vi "Split Registers by Direction.vi"(7 "Group":bool, 8 "error in":errorcluster, 11 "vi info":T1 {"RegisterMap"."Address" format="%.0x"}) -> (0 "error out":errorcluster, 2 "Controls":T8[](array[typedef]) {"Data Type" format="%.0x"}, 3 "Indicator":T8[](array[typedef]) {"Data Type" format="%.0x"})   [LabVIEW 2018, in "FPGA Addon System Explorer.lvlib"]
uses:
  FPGA Addon System Explorer.lvlib
  Addon Shared/Types/Register Information.ctl
  Addon Shared/Types/Data Type.ctl
  <vilib>/rvi/Bitfile/niFpgaBitfileStructure_VI.ctl
  <vilib>/rvi/Bitfile/nirviControlStructure.ctl
  <vilib>/rvi/Bitfile/nirviTypdefDescription.ctl
  <vilib>/rvi/Bitfile/nirviMechanicalAction.ctl
  <vilib>/rvi/Bitfile/nirviSubControlStructure.ctl
  <vilib>/rvi/Bitfile/nirviClusterElementControl.ctl
  <vilib>/picture/picture.llb/imagedata.ctl
  niveristand-fpga-addon-speciality-io/Source/Types/PWM.Measure.Analog.Measurement.ctl
  niveristand-fpga-addon-speciality-io/Source/Types/PWM.Measure.Digital.Measurement.ctl
  niveristand-fpga-addon-speciality-io/Source/Types/Static.Measure.Digital.Measurement.ctl
  niveristand-fpga-addon-speciality-io/Source/Types/QuadratureEncoder.Measure.Digital.Measurement.ctl
  niveristand-fpga-addon-speciality-io/Source/Types/PWM.Generate.Digital.Settings.ctl
  niveristand-fpga-addon-speciality-io/Source/Types/PWM.Measure.Analog.Settings.ctl
  niveristand-fpga-addon-speciality-io/Source/Types/PWM.Measure.Digital.Settings.ctl
  niveristand-fpga-addon-speciality-io/Source/Types/Sine.Generate.Settings.ctl
  niveristand-fpga-addon-speciality-io/Source/Types/Static.Generate.Digital.Settings.ctl
  niveristand-fpga-addon-speciality-io/Source/Types/Static.Measure.Digital.Settings.ctl
  niveristand-fpga-addon-speciality-io/Source/Types/WSS.Generate.Digital.Settings.ctl
  niveristand-fpga-addon-speciality-io/Source/Types/QuadratureEncoder.Measure.Digital.Settings.ctl
  Addon Shared/FPGA Addon Shared.lvlib
  niveristand-fpga-addon-speciality-io/Source/Speciality FPGA IO.lvlib
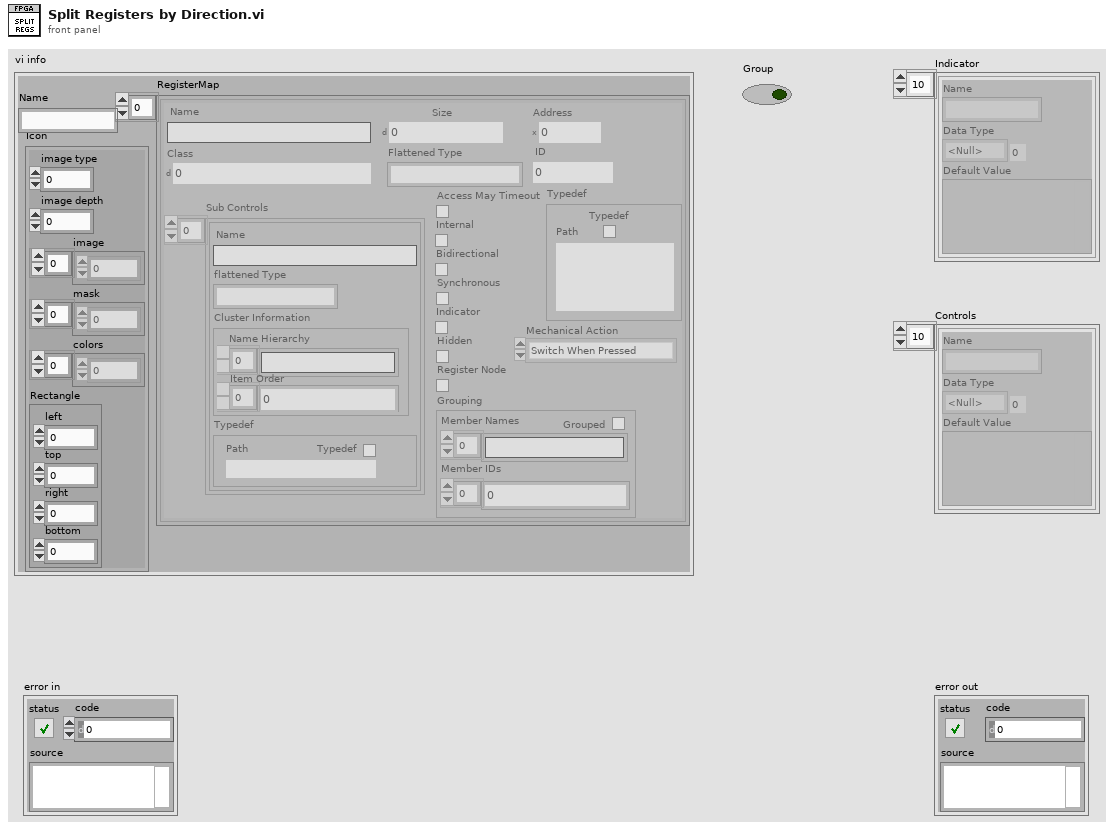
[diagram p1: front panel]
types:
  T1 = typedef "niFpgaBitfileStructure_VI.ctl" = cluster{"Name":string, "RegisterMap":T2[], "Icon":T7}
  T2 = typedef "nirviControlStructure.ctl" = cluster{"Name":string, "Hidden":bool, "Indicator":bool, "Flattened Type":string, "Grouping":cluster{"Grouped":bool, "Member Names":string[], "Member IDs":u32[]}, "Address":u32, "Size":u32, "Class":u32, "Internal":bool, "Typedef":T3, "ID":u32, "Bidirectional":bool, "Synchronous":bool, "Mechanical Action":T4, "Sub Controls":T5[], "Access May Timeout":bool, "Register Node":bool}
  T3 = typedef "nirviTypdefDescription.ctl" = cluster{"Typedef":bool, "Path":path}
  T4 = typedef "nirviMechanicalAction.ctl" = enum8{"Switch When Pressed", "Switch When Released", "Switch Until Released", "Latch When Pressed", "Latch When Released", "Latch Until Released"}
  T5 = typedef "nirviSubControlStructure.ctl" = cluster{"Name":string, "flattened Type":string, "Cluster Information":T6, "Typedef":T3}
  T6 = typedef "nirviClusterElementControl.ctl" = cluster{"Name Hierarchy":string[], "Item Order":u32[]}
  T7 = typedef "imagedata.ctl" = cluster{"image type":i32, "image depth":i32, "image":u8[], "mask":u8[], "colors":u32[], "Rectangle":cluster{"left":i16, "top":i16, "right":i16, "bottom":i16}}
  T8 = typedef "FPGA Addon Shared.lvlib/Register Information.ctl" = cluster{"Name":string, "Data Type":T9, "Default Value":variant}
  T9 = typedef "FPGA Addon Shared.lvlib/Data Type.ctl" = enum8{"<Null>", "I8", "I16", "I32", "I64", "U8", "U16", "U32", "U64", "SGL", "Boolean", "Analog PWM In Settings", "Analog PWM In", "Digital PWM In Settings", "Digital PWM In", "Digital PWM Out", "Sine Out", "FXP+/-24.5", "FXP+/-16.5", "FXP+/-32.8", "FXP+/-64.32", "FXP+/-16.7", "FXP+/-20.5", "FXP+/-27.5", "FXP+/-32.16", "FXP+16.3", "FXP+18.3", "Digital Static In", "Digital Static Out", "Digital Static In Settings", "Digital WSS Out", "Quad Encoder Settings", "Quad Encoder In", "Group"}
  T10 = typedef "Speciality FPGA IO.lvlib/QuadratureEncoder.Measure.Digital.Measurement.ctl" = cluster{"POSITION":i32}
  T11 = typedef "Speciality FPGA IO.lvlib/Static.Measure.Digital.Measurement.ctl" = cluster{"STATE":bool}
  T12 = typedef "Speciality FPGA IO.lvlib/PWM.Measure.Digital.Measurement.ctl" = cluster{"ACTIVE TICKS":u32, "INACTIVE TICKS":u32, "ACQ TICKS":u32}
  T13 = typedef "Speciality FPGA IO.lvlib/PWM.Measure.Analog.Measurement.ctl" = cluster{"ACTIVE TICKS":u32, "INACTIVE TICKS":u32, "ACQ TICKS":u32, "ACTIVE VOLTAGE":fxp<+/-,32,8>, "INACTIVE VOLTAGE":fxp<+/-,32,8>}
  T14 = typedef "Speciality FPGA IO.lvlib/QuadratureEncoder.Measure.Digital.Settings.ctl" = cluster{"DIRECTION":u8, "RESET VALUE":i32, "A RESET STATE":bool, "B RESET STATE":bool, "Z RESET STATE":bool}
  T15 = typedef "Speciality FPGA IO.lvlib/WSS.Generate.Digital.Settings.ctl" = cluster{"ACTIVE EDGE":bool, "ACTIVE TICKS":u32, "INACTIVE TICKS":u32, "DATA":u8, "SENSOR TYPE":u8}
  T16 = typedef "Speciality FPGA IO.lvlib/Static.Measure.Digital.Settings.ctl" = cluster{"ACTIVE EDGE":bool}
  T17 = typedef "Speciality FPGA IO.lvlib/Static.Generate.Digital.Settings.ctl" = cluster{"ACTIVE EDGE":bool, "OUTPUT":bool}
  T18 = typedef "Speciality FPGA IO.lvlib/Sine.Generate.Settings.ctl" = cluster{"AMP":fxp<+/-,32,8>, "OFFSET":fxp<+/-,32,8>, "PERIODS/TICKS":fxp<+,32,0>}
  T19 = typedef "Speciality FPGA IO.lvlib/PWM.Measure.Digital.Settings.ctl" = cluster{"ACTIVE EDGE":bool, "TIMEOUT":u32}
  T20 = typedef "Speciality FPGA IO.lvlib/PWM.Measure.Analog.Settings.ctl" = cluster{"ACTIVE EDGE":bool, "TIMEOUT":u32, "THRESHOLD":fxp<+/-,32,8>}
  T21 = typedef "Speciality FPGA IO.lvlib/PWM.Generate.Digital.Settings.ctl" = cluster{"ACTIVE EDGE":bool, "ACTIVE TICKS":u32, "INACTIVE TICKS":u32}
  T22 = typedef "Type Descriptor Enumeration__ogtk.ctl" = enum8{"<Null>", "I8", "I16", "I32", "I64", "U8", "U16", "U32", "U64", "SGL", "DBL", "EXT", "CSG", "CDB", "CXT", "0x0F", "0x10", "0x11", "0x12", "0x13", "0x14", "Enum U8", "Enum U16", "Enum U32", "Enum U64", "SGL PQ", "DBL PQ", "EXT PQ", "CSG PQ", "CDB PQ", "CXT PQ", "0x1F", "0x20", "Boolean", "0x22", "0x23", "0x24", "0x25", "0x26", "0x27", "0x28", "0x29", "0x2A", "0x2B", "0x2C", "0x2D", "0x2E", "0x2F", "String", "0x31", "Path", "Pict", "0x34", "0x35", "0x36", "DAQ", "0x38", "0x39", "0x3A", "0x3B", "0x3C", "0x3D", "0x3E", "0x3F", "Array", "0x41", "0x42", "0x43", "0x44", "0x45", "0x46", "0x47", "0x48", "0x49", "0x4A", "0x4B", "0x4C", "0x4D", "0x4E", "0x4F", "Cluster", "0x51", "0x52", "Variant", "Waveform", "0x55", "0x56", "0x57", "0x58", "0x59", "0x5A", "0x5B", "0x5C", "0x5D", "0x5E", "0x5F", "0x60", "0x61", "0x62", "0x63", "0x64", "0x65", "0x66", "0x67", "0x68", "0x69", "0x6A", "0x6B", "0x6C", "0x6D", "0x6E", "0x6F", "Refnum"}
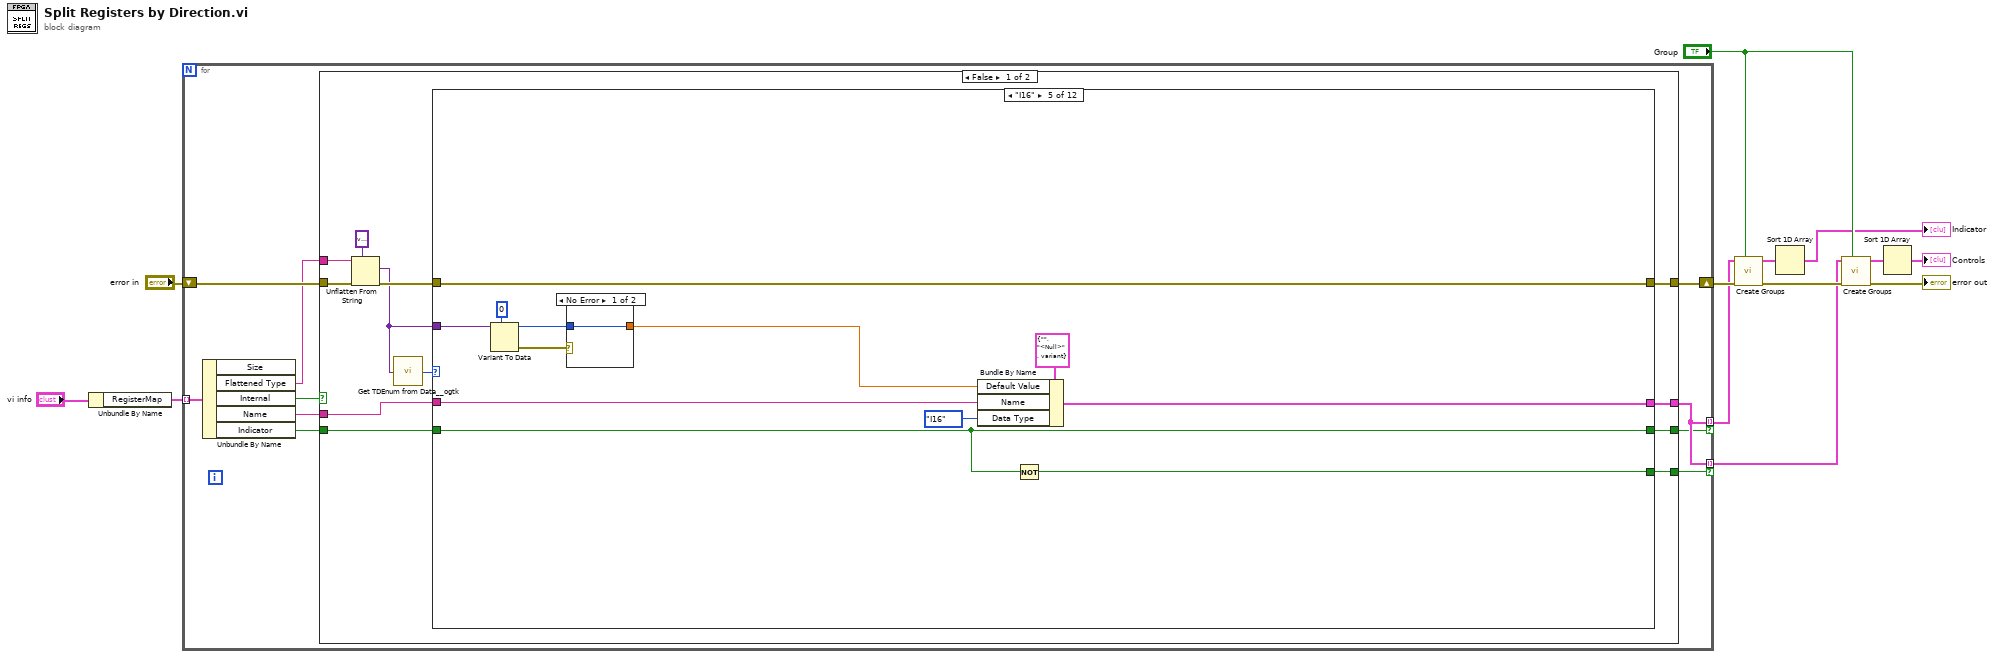
[diagram p0: block diagram]
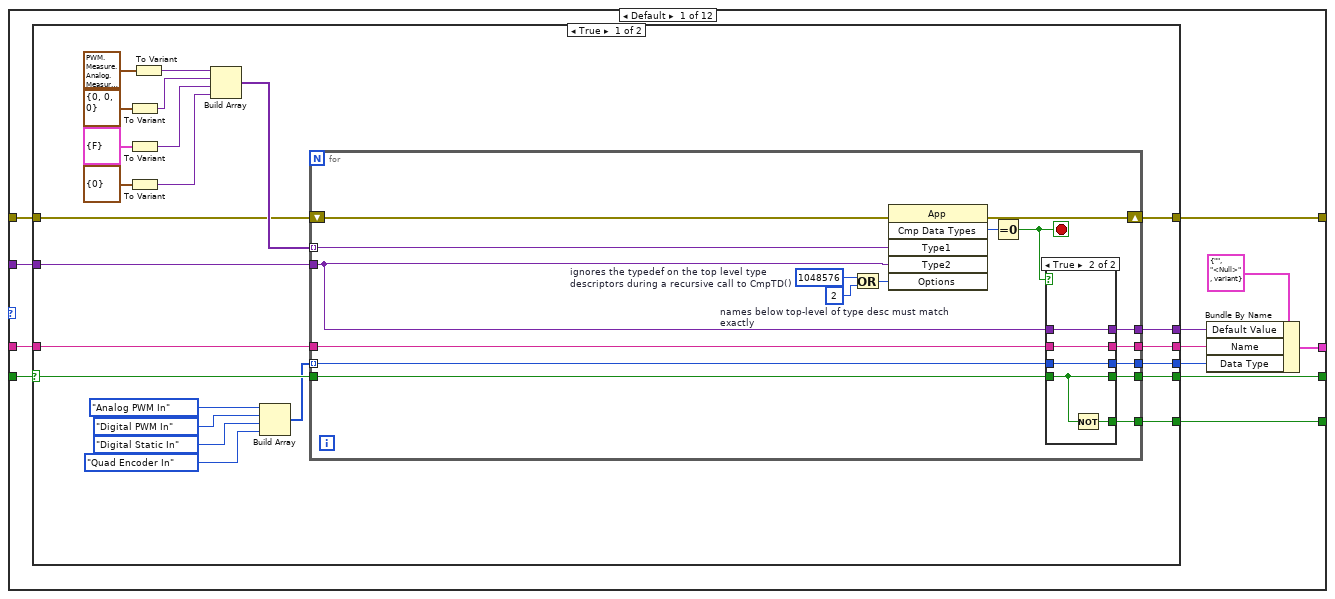
[diagram p2: hidden frame]
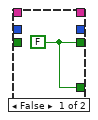
[diagram p3: hidden frame]
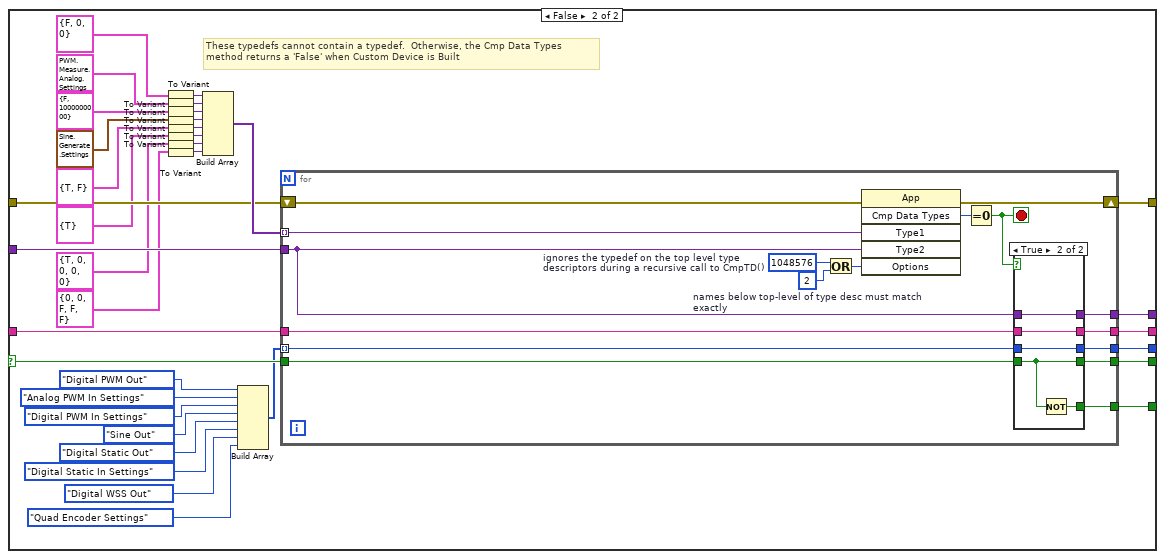
[diagram p4: hidden frame]
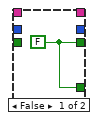
[diagram p5: hidden frame]
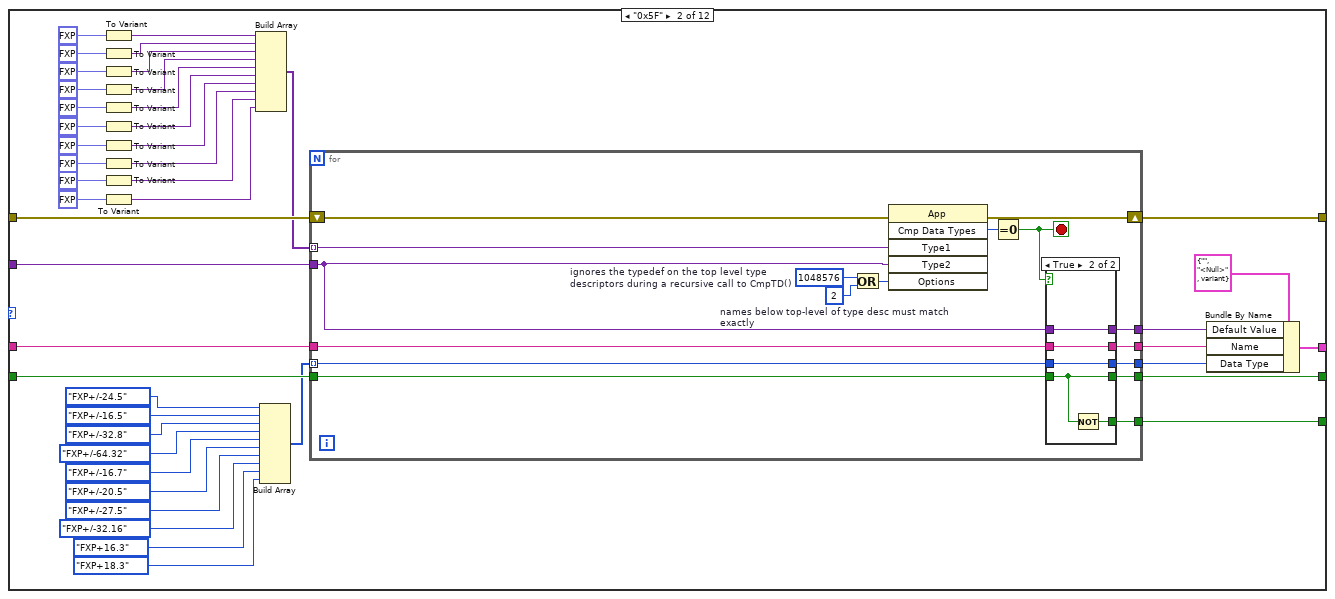
[diagram p6: hidden frame]
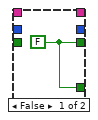
[diagram p7: hidden frame]
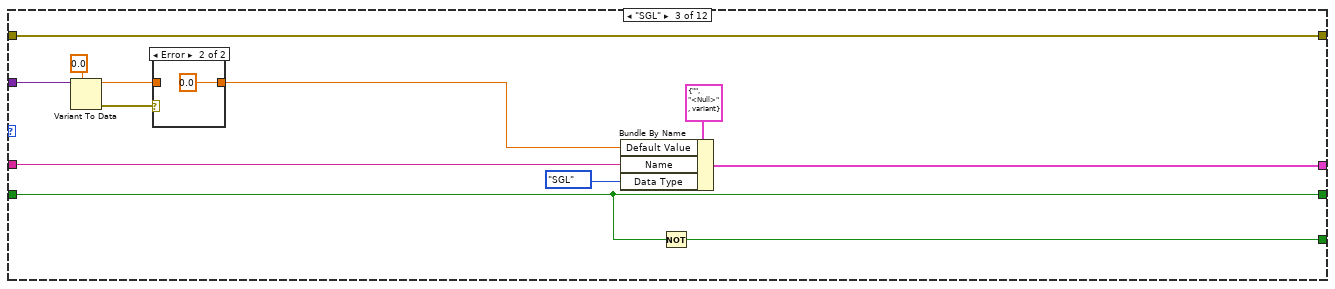
[diagram p8: hidden frame]
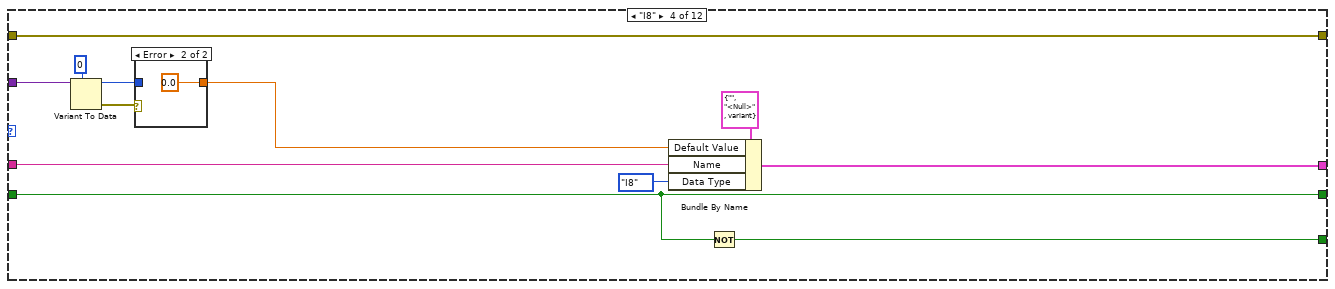
[diagram p10: hidden frame]
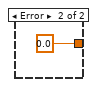
[diagram p12: hidden frame]
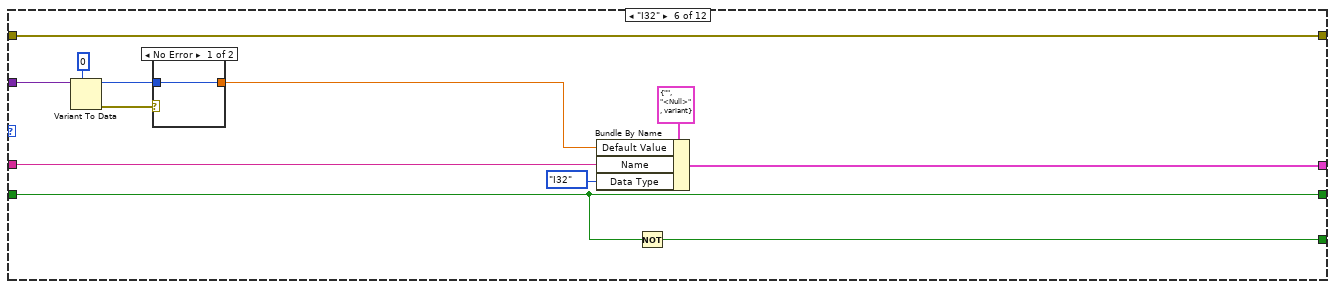
[diagram p13: hidden frame]
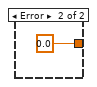
[diagram p14: hidden frame]
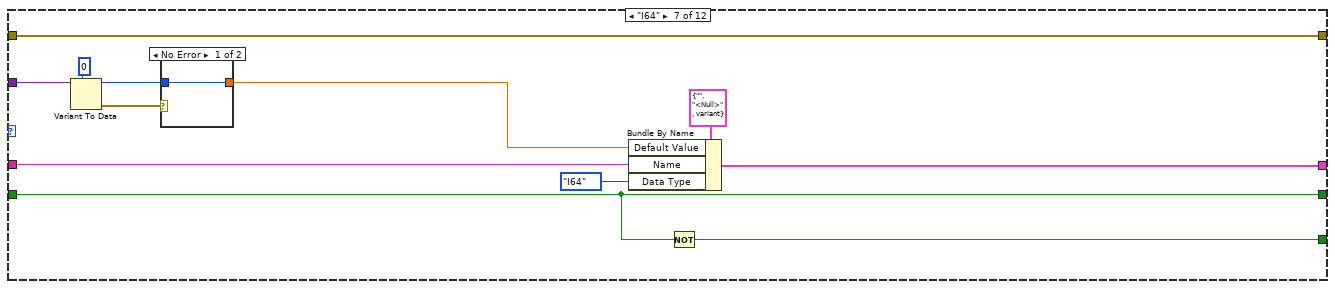
[diagram p15: hidden frame]
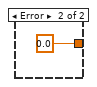
[diagram p16: hidden frame]
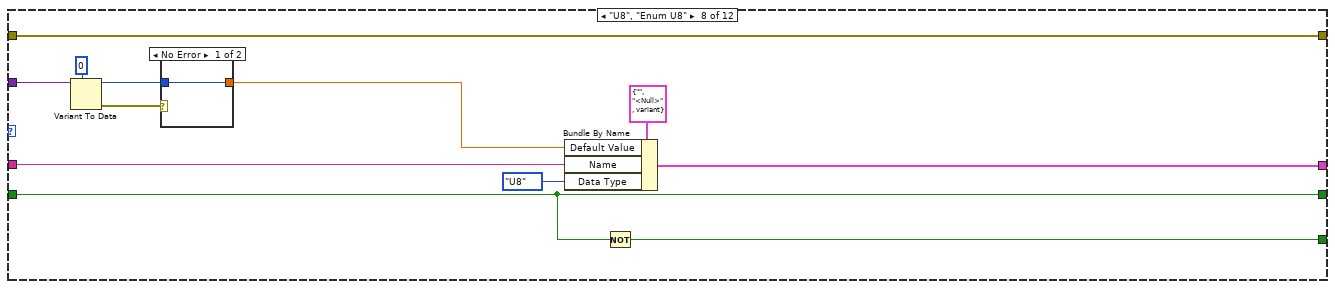
[diagram p17: hidden frame]
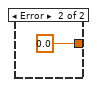
[diagram p18: hidden frame]
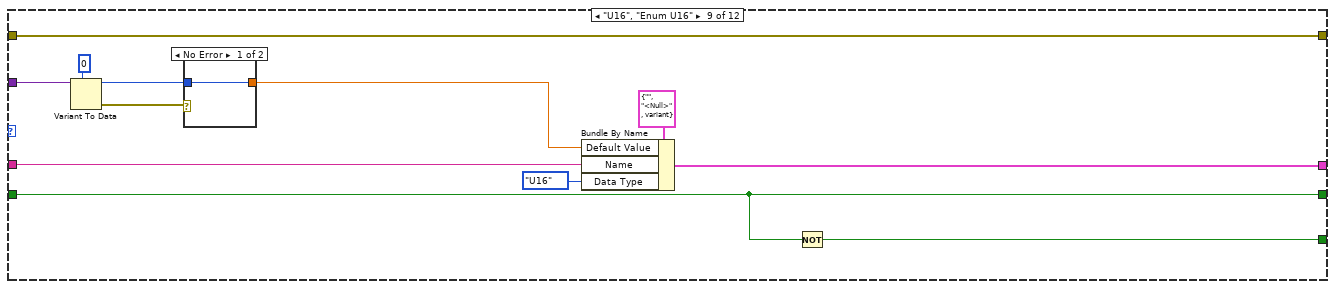
[diagram p19: hidden frame]
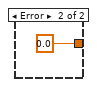
[diagram p20: hidden frame]
diagram:
  n1 = Unbundle By Name("vi info") -> ("RegisterMap"=w13:T2[])
  n2 = for {
    tunnel: w13 -> [w18] mode=indexing
    tunnel: [w23] -> w6 mode=indexing if=w22
    tunnel: [w23] -> w5 mode=indexing if=w21
    shift-right: [w20] -> w10
    shift-left: "error in" -> [w19]
    n3 = Unbundle By Name(w18) -> ("Flattened Type"=w14:string, "Internal"=w15:bool, "Name"=w16:string, "Indicator"=w17:bool)  [unwired: 1 out]
    n4 = case shown="False" w15 {
      tunnel: w16 -> [w34 _]
      tunnel: w17 -> [w33 _]
      tunnel: [w32 _] -> w23
      tunnel: [w31 w363] -> w22
      tunnel: [w30 w363] -> w21
      tunnel: w14 -> [w27 _]
      tunnel: [w29 w362] -> w20
      tunnel: w19 -> [w26 w362]
      frame False {
        n5 = Unflatten From String(type=variant ("Variant"), binary string=w27, error in (no error)=w26) -> (value=w24:variant, error out=w25:errorcluster)  [unwired: 3 out]
        n6 = call <userlib>:"Get TDEnum from Data__ogtk.vi"("Data"=w24) -> ("Type Descriptor Enumeration"=w35:T22)  [unwired: 4 in]
        n7 = case shown="\"I16\"" w35 {
          tunnel: [w47 w197 w229 w243 w257 w271 w285 w299 w313 w327 w341 w355] -> w31
          tunnel: w33 -> [w42 w192 w229 w243 w257 w271 w285 w299 w313 w327 w341 w355]
          tunnel: w34 -> [w43 w193 w231 w245 w259 w273 w287 w301 w315 w329 w343 w357]
          tunnel: [w44 w194 w230 w244 w258 w272 w286 w300 w314 w328 w342 w356] -> w32
          tunnel: [w46 w196 w228 w242 w256 w270 w284 w298 w312 w326 w340 w354] -> w30
          tunnel: w24 -> [w41 w191 w227 w241 w255 w269 w283 w297 w311 w325 w339 w353]
          tunnel: [w37 w187 w221 w235 w249 w263 w277 w291 w305 w319 w333 w347] -> w29
          tunnel: w25 -> [w36 w186 w221 w235 w249 w263 w277 w291 w305 w319 w333 w347]
          frame Default {
            n8 = case shown="True" w42 {
              selector: w42 -> [w66 w126]
              tunnel: [w71 w130] -> w47
              tunnel: [w70 w129] -> w46
              tunnel: w43 -> [w69 w128]
              tunnel: w41 -> [w60 w122]
              tunnel: [w59 w121] -> w40
              tunnel: [w58 w120] -> w39
              tunnel: [w57 w119] -> w38
              tunnel: [w55 w110] -> w37
              tunnel: w36 -> [w54 w111]
              frame True {
                n9 = To Variant(anything=T12 {"ACTIVE TICKS"=0, "INACTIVE TICKS"=0, "ACQ TICKS"=0} ("Cached.Data")) -> (Variant=w64:variant)
                n10 = To Variant(anything=T11 {"STATE"=FALSE} ("Cached.Data")) -> (Variant=w52:variant)
                n11 = To Variant(anything=T10 {"POSITION"=0} ("Cached.Data")) -> (Variant=w48:variant)
                n12 = To Variant(anything=T13 {"ACTIVE TICKS"=0, "INACTIVE TICKS"=0, "ACQ TICKS"=0, "ACTIVE VOLTAGE"=0.0, "INACTIVE VOLTAGE"=0.0} ("Cached.Data")) -> (Variant=w65:variant)
                n13 = Build Array(w65, w64, w52, w48) -> (w61:variant[])
                n14 = Build Array(Data_Type."Analog PWM In" ("Data Type"), Data_Type."Digital PWM In" ("Data Type"), Data_Type."Digital Static In" ("Data Type"), Data_Type."Quad Encoder In" ("Data Type")) -> (w56:T9[])
                n15 = for {
                  tunnel: w60 -> [w75]
                  tunnel: [w86] -> w70
                  tunnel: w69 -> [w85]
                  tunnel: w61 -> [w77] mode=indexing
                  tunnel: [w84] -> w58
                  tunnel: [w83] -> w59
                  tunnel: [w82] -> w57
                  tunnel: w56 -> [w81] mode=indexing
                  tunnel: w66 -> [w88]
                  tunnel: [w87] -> w71
                  shift-right: [w72] -> w55
                  shift-left: w54 -> [w73]
                  stop <- w76 stop-if-true
                  w74 = 2  # names below top-level of type desc must match exactly
                  w79 = 1048576  # ignores the typedef on the top level type descriptors during a recursive call to CmpTD()
                  n16 = Or(x=w79, y=w74) -> (x .or. y?=w80:i32)
                  n17 = invoke class="App" method="Cmp Data Types"(error in=w73, "Type1"=w77, "Type2"=w75, "Options"=w80) -> (error out=w72:errorcluster, "Compare Data Types"=w78:i32)  [unwired: 2 in, 4 out]
                  n18 = Equal To 0?(x=w78) -> (x = 0?=w76:bool)
                  n19 = case shown="True" w76 {
                    tunnel: w88 -> [_ w94]
                    tunnel: [w89 w94] -> w87
                    tunnel: [w89 w93] -> w86
                    tunnel: w85 -> [_ w91]
                    tunnel: [_ w92] -> w84
                    tunnel: w75 -> [_ w92]
                    tunnel: [_ w91] -> w83
                    tunnel: [_ w90] -> w82
                    tunnel: w81 -> [_ w90]
                    frame False {
                      w89 = FALSE ("Boolean")
                    }
                    frame True {
                      n20 = Not(x=w94) -> (.not. x?=w93:bool)
                    }
                  }
                }
              }
              frame False {
                # "These typedefs cannot contain a typedef.  Otherwise, the Cmp Data Types \nmethod returns a 'False' when Custom Device is Built"
                n21 = To Variant(anything=T21 {"ACTIVE EDGE"=FALSE, "ACTIVE TICKS"=0, "INACTIVE TICKS"=0} ("Channel.Settings")) -> (Variant=w125:variant)
                n22 = To Variant(anything=T20 {"ACTIVE EDGE"=FALSE, "TIMEOUT"=1000000000, "THRESHOLD"=3.0} ("Channel.Settings")) -> (Variant=w115:variant)
                n23 = To Variant(anything=T19 {"ACTIVE EDGE"=FALSE, "TIMEOUT"=1000000000} ("Channel.Settings")) -> (Variant=w114:variant)
                n24 = To Variant(anything=T18 {"AMP"=0.0, "OFFSET"=0.0, "PERIODS/TICKS"=0.0002500000409781933} ("Settings")) -> (Variant=w108:variant)
                n25 = To Variant(anything=T17 {"ACTIVE EDGE"=TRUE, "OUTPUT"=FALSE} ("Settings")) -> (Variant=w106:variant)
                n26 = To Variant(anything=T16 {"ACTIVE EDGE"=TRUE} ("Settings")) -> (Variant=w103:variant)
                n27 = To Variant(anything=T15 {"ACTIVE EDGE"=TRUE, "ACTIVE TICKS"=0, "INACTIVE TICKS"=0, "DATA"=0, "SENSOR TYPE"=0} ("Wheel Speed Sensor Settings")) -> (Variant=w99:variant)
                n28 = To Variant(anything=T14 {"DIRECTION"=0, "RESET VALUE"=0, "A RESET STATE"=FALSE, "B RESET STATE"=FALSE, "Z RESET STATE"=FALSE} ("Settings")) -> (Variant=w96:variant)
                n29 = Build Array(w125, w115, w114, w108, w106, w103, w99, w96) -> (w123:variant[])
                n30 = Build Array(Data_Type."Digital PWM Out" ("Data Type"), Data_Type."Analog PWM In Settings" ("Data Type"), Data_Type."Digital PWM In Settings" ("Data Type"), Data_Type."Sine Out" ("Data Type"), Data_Type."Digital Static Out" ("Data Type"), Data_Type."Digital Static In Settings" ("Data Type"), Data_Type."Digital WSS Out" ("Data Type"), Data_Type."Quad Encoder Settings" ("Data Type")) -> (w118:T9[])
                n31 = for {
                  tunnel: w122 -> [w136]
                  tunnel: [w145] -> w129
                  tunnel: w128 -> [w144]
                  tunnel: w123 -> [w135] mode=indexing
                  tunnel: [w143] -> w120
                  tunnel: [w142] -> w121
                  tunnel: [w141] -> w119
                  tunnel: w118 -> [w140] mode=indexing
                  tunnel: w126 -> [w147]
                  tunnel: [w146] -> w130
                  shift-right: [w131] -> w110
                  shift-left: w111 -> [w132]
                  stop <- w133 stop-if-true
                  w138 = 2  # names below top-level of type desc must match exactly
                  w137 = 1048576  # ignores the typedef on the top level type descriptors during a recursive call to CmpTD()
                  n32 = Or(x=w137, y=w138) -> (x .or. y?=w139:i32)
                  n33 = invoke class="App" method="Cmp Data Types"(error in=w132, "Type1"=w135, "Type2"=w136, "Options"=w139) -> (error out=w131:errorcluster, "Compare Data Types"=w134:i32)  [unwired: 2 in, 4 out]
                  n34 = Equal To 0?(x=w134) -> (x = 0?=w133:bool)
                  n35 = case shown="True" w133 {
                    tunnel: w147 -> [_ w153]
                    tunnel: [w148 w153] -> w146
                    tunnel: [w148 w152] -> w145
                    tunnel: w144 -> [_ w150]
                    tunnel: [_ w151] -> w143
                    tunnel: w136 -> [_ w151]
                    tunnel: [_ w150] -> w142
                    tunnel: [_ w149] -> w141
                    tunnel: w140 -> [_ w149]
                    frame False {
                      w148 = FALSE ("Boolean")
                    }
                    frame True {
                      n36 = Not(x=w153) -> (.not. x?=w152:bool)
                    }
                  }
                }
              }
            }
            n37 = Bundle By Name(cluster=T8 {"Name"="", "Data Type"=enum."<Null>", "Default Value"=variant(refnum<class> refnum)}, "Default Value"=w39, "Name"=w40, "Data Type"=w38) -> (w44:T8)
          }
          frame "0x5F" {
            n38 = To Variant(anything=fxp<+/-,24,5> 0.0 ("Numeric 1 In")) -> (Variant=w185:variant)
            n39 = To Variant(anything=fxp<+/-,16,5> 0.0 ("Numeric 2 In")) -> (Variant=w184:variant)
            n40 = To Variant(anything=fxp<+/-,32,8> 0.0 ("Numeric 3 In")) -> (Variant=w177:variant)
            n41 = To Variant(anything=fxp<+/-,64,32> 0.0 ("Numeric 4 In")) -> (Variant=w176:variant)
            n42 = To Variant(anything=fxp<+/-,16,7> 0.0 ("Numeric 4 In")) -> (Variant=w170:variant)
            n43 = To Variant(anything=fxp<+/-,20,5> 0.0 ("Numeric 4 In")) -> (Variant=w167:variant)
            n44 = To Variant(anything=fxp<+/-,27,5> 0.0 ("Numeric 4 In")) -> (Variant=w164:variant)
            n45 = To Variant(anything=fxp<+/-,32,16> 0.0 ("Numeric 4 In")) -> (Variant=w161:variant)
            n46 = To Variant(anything=fxp<+,16,3> 0.0 ("Numeric 4 In")) -> (Variant=w158:variant)
            n47 = To Variant(anything=fxp<+,18,3> 0.0 ("Numeric 4 In")) -> (Variant=w156:variant)
            n48 = Build Array(w185, w184, w177, w176, w170, w167, w164, w161, w158, w156) -> (w181:variant[])
            n49 = Build Array(Data_Type."FXP+/-24.5" ("Data Type"), Data_Type."FXP+/-16.5" ("Data Type"), Data_Type."FXP+/-32.8" ("Data Type"), Data_Type."FXP+/-64.32" ("Data Type"), Data_Type."FXP+/-16.7" ("Data Type"), Data_Type."FXP+/-20.5" ("Data Type"), Data_Type."FXP+/-27.5" ("Data Type"), Data_Type."FXP+/-32.16" ("Data Type"), Data_Type."FXP+16.3" ("Data Type"), Data_Type."FXP+18.3" ("Data Type")) -> (w180:T9[])
            n50 = for {
              tunnel: w191 -> [w201]
              tunnel: [w212] -> w196
              tunnel: w193 -> [w211]
              tunnel: w181 -> [w203] mode=indexing
              tunnel: [w210] -> w189
              tunnel: [w209] -> w190
              tunnel: [w208] -> w188
              tunnel: w180 -> [w207] mode=indexing
              tunnel: w192 -> [w214]
              tunnel: [w213] -> w197
              shift-right: [w198] -> w187
              shift-left: w186 -> [w199]
              stop <- w202 stop-if-true
              w200 = 2  # names below top-level of type desc must match exactly
              w205 = 1048576  # ignores the typedef on the top level type descriptors during a recursive call to CmpTD()
              n51 = Or(x=w205, y=w200) -> (x .or. y?=w206:i32)
              n52 = invoke class="App" method="Cmp Data Types"(error in=w199, "Type1"=w203, "Type2"=w201, "Options"=w206) -> (error out=w198:errorcluster, "Compare Data Types"=w204:i32)  [unwired: 2 in, 4 out]
              n53 = Equal To 0?(x=w204) -> (x = 0?=w202:bool)
              n54 = case shown="True" w202 {
                tunnel: w214 -> [_ w220]
                tunnel: [w215 w220] -> w213
                tunnel: [w215 w219] -> w212
                tunnel: w211 -> [_ w217]
                tunnel: [_ w218] -> w210
                tunnel: w201 -> [_ w218]
                tunnel: [_ w217] -> w209
                tunnel: [_ w216] -> w208
                tunnel: w207 -> [_ w216]
                frame False {
                  w215 = FALSE ("Boolean")
                }
                frame True {
                  n55 = Not(x=w220) -> (.not. x?=w219:bool)
                }
              }
            }
            n56 = Bundle By Name(cluster=T8 {"Name"="", "Data Type"=enum."<Null>", "Default Value"=variant(refnum<class> refnum)}, "Default Value"=w189, "Name"=w190, "Data Type"=w188) -> (w194:T8)
          }
          frame "SGL" {
            n57 = Variant To Data(type=sgl 0.0, Variant=w227) -> (data=w223:sgl, error out=w225:errorcluster)  [unwired: 1 in]
            n58 = case shown="Error" w225 {
              tunnel: [w233 0.0] -> w224
              tunnel: w223 -> [w233 _]
              frame No Error {
              }
              frame Error {
              }
            }
            n59 = Bundle By Name(cluster=T8 {"Name"="", "Data Type"=enum."<Null>", "Default Value"=variant(refnum<class> refnum)}, "Default Value"=w224, "Name"=w231, "Data Type"=Data_Type."SGL") -> (w230:T8)
            n60 = Not(x=w229) -> (.not. x?=w228:bool)
          }
          frame "I8" {
            n61 = Variant To Data(type=i8 0, Variant=w241) -> (data=w237:i8, error out=w239:errorcluster)  [unwired: 1 in]
            n62 = case shown="Error" w239 {
              tunnel: [w247 0.0] -> w238
              tunnel: w237 -> [w247 _]
              frame No Error {
              }
              frame Error {
              }
            }
            n63 = Bundle By Name(cluster=T8 {"Name"="", "Data Type"=enum."<Null>", "Default Value"=variant(refnum<class> refnum)}, "Default Value"=w238, "Name"=w245, "Data Type"=Data_Type."I8") -> (w244:T8)
            n64 = Not(x=w243) -> (.not. x?=w242:bool)
          }
          frame "I16" {
            n65 = Variant To Data(type=i16 0, Variant=w255) -> (data=w251:i16, error out=w253:errorcluster)  [unwired: 1 in]
            n66 = case shown="No Error" w253 {
              tunnel: [w261 0.0] -> w252
              tunnel: w251 -> [w261 _]
              frame No Error {
              }
              frame Error {
              }
            }
            n67 = Bundle By Name(cluster=T8 {"Name"="", "Data Type"=enum."<Null>", "Default Value"=variant(refnum<class> refnum)}, "Default Value"=w252, "Name"=w259, "Data Type"=Data_Type."I16") -> (w258:T8)
            n68 = Not(x=w257) -> (.not. x?=w256:bool)
          }
          frame "I32" {
            n69 = Variant To Data(type=0, Variant=w269) -> (data=w265:i32, error out=w267:errorcluster)  [unwired: 1 in]
            n70 = case shown="No Error" w267 {
              tunnel: [w275 0.0] -> w266
              tunnel: w265 -> [w275 _]
              frame No Error {
              }
              frame Error {
              }
            }
            n71 = Bundle By Name(cluster=T8 {"Name"="", "Data Type"=enum."<Null>", "Default Value"=variant(refnum<class> refnum)}, "Default Value"=w266, "Name"=w273, "Data Type"=Data_Type."I32") -> (w272:T8)
            n72 = Not(x=w271) -> (.not. x?=w270:bool)
          }
          frame "I64" {
            n73 = Variant To Data(type=i64 0, Variant=w283) -> (data=w279:i64, error out=w281:errorcluster)  [unwired: 1 in]
            n74 = case shown="No Error" w281 {
              tunnel: [w289 0.0] -> w280
              tunnel: w279 -> [w289 _]
              frame No Error {
              }
              frame Error {
              }
            }
            n75 = Bundle By Name(cluster=T8 {"Name"="", "Data Type"=enum."<Null>", "Default Value"=variant(refnum<class> refnum)}, "Default Value"=w280, "Name"=w287, "Data Type"=Data_Type."I64") -> (w286:T8)
            n76 = Not(x=w285) -> (.not. x?=w284:bool)
          }
          frame "U8", "Enum U8" {
            n77 = Variant To Data(type=u8 0, Variant=w297) -> (data=w293:u8, error out=w295:errorcluster)  [unwired: 1 in]
            n78 = case shown="No Error" w295 {
              tunnel: [w303 0.0] -> w294
              tunnel: w293 -> [w303 _]
              frame No Error {
              }
              frame Error {
              }
            }
            n79 = Bundle By Name(cluster=T8 {"Name"="", "Data Type"=enum."<Null>", "Default Value"=variant(refnum<class> refnum)}, "Default Value"=w294, "Name"=w301, "Data Type"=Data_Type."U8") -> (w300:T8)
            n80 = Not(x=w299) -> (.not. x?=w298:bool)
          }
          frame "U16", "Enum U16" {
            n81 = Variant To Data(type=u16 0, Variant=w311) -> (data=w307:u16, error out=w309:errorcluster)  [unwired: 1 in]
            n82 = case shown="No Error" w309 {
              tunnel: [w317 0.0] -> w308
              tunnel: w307 -> [w317 _]
              frame No Error {
              }
              frame Error {
              }
            }
            n83 = Bundle By Name(cluster=T8 {"Name"="", "Data Type"=enum."<Null>", "Default Value"=variant(refnum<class> refnum)}, "Default Value"=w308, "Name"=w315, "Data Type"=Data_Type."U16") -> (w314:T8)
            n84 = Not(x=w313) -> (.not. x?=w312:bool)
          }
          frame "U32", "Enum U32" {
            n85 = Variant To Data(type=u32 0, Variant=w325) -> (data=w321:u32, error out=w323:errorcluster)  [unwired: 1 in]
            n86 = case shown="No Error" w323 {
              tunnel: [w331 0.0] -> w322
              tunnel: w321 -> [w331 _]
              frame No Error {
              }
              frame Error {
              }
            }
            n87 = Bundle By Name(cluster=T8 {"Name"="", "Data Type"=enum."<Null>", "Default Value"=variant(refnum<class> refnum)}, "Default Value"=w322, "Name"=w329, "Data Type"=Data_Type."U32") -> (w328:T8)
            n88 = Not(x=w327) -> (.not. x?=w326:bool)
          }
          frame "U64", "Enum U64" {
            n89 = Variant To Data(type=u64 0, Variant=w339) -> (data=w335:u64, error out=w337:errorcluster)  [unwired: 1 in]
            n90 = case shown="No Error" w337 {
              tunnel: [w345 0.0] -> w336
              tunnel: w335 -> [w345 _]
              frame No Error {
              }
              frame Error {
              }
            }
            n91 = Bundle By Name(cluster=T8 {"Name"="", "Data Type"=enum."<Null>", "Default Value"=variant(refnum<class> refnum)}, "Default Value"=w336, "Name"=w343, "Data Type"=Data_Type."U64") -> (w342:T8)
            n92 = Not(x=w341) -> (.not. x?=w340:bool)
          }
          frame "Boolean" {
            n93 = Variant To Data(type=FALSE, Variant=w353) -> (data=w349:bool, error out=w351:errorcluster)  [unwired: 1 in]
            n94 = case shown="No Error" w351 {
              tunnel: [w359 0.0] -> w350
              tunnel: w349 -> [w360 _]
              frame No Error {
                n95 = Boolean To (0,1)(Boolean=w360) -> (0, 1=w359:i16)
              }
              frame Error {
              }
            }
            n96 = Bundle By Name(cluster=T8 {"Name"="", "Data Type"=enum."<Null>", "Default Value"=variant(refnum<class> refnum)}, "Default Value"=w350, "Name"=w357, "Data Type"=Data_Type."Boolean") -> (w356:T8)
            n97 = Not(x=w355) -> (.not. x?=w354:bool)
          }
        }
      }
      frame True {
        w363 = FALSE ("Boolean")
      }
    }
  }
  n98 = call "Create Groups.vi"("Group"="Group", "error in (no error)"=w10, "Channels"=w6) -> ("error out"=w9:errorcluster, "Channels out"=w4:T8[])  [unwired: 7 in]
  n99 = Sort 1D Array(array=w4) -> (sorted array=→"Indicator":T8[])
  n100 = call "Create Groups.vi"("Group"="Group", "error in (no error)"=w9, "Channels"=w5) -> ("error out"=→"error out":errorcluster, "Channels out"=w2:T8[])  [unwired: 7 in]
  n101 = Sort 1D Array(array=w2) -> (sorted array=→"Controls":T8[])
